vi "TCL Open BaseFile.vi"() -> (0 "error out":errorcluster, 1 "Event File Refnum":refnum<k1>)   [LabVIEW 2009]
uses:
  TCL Global.vi
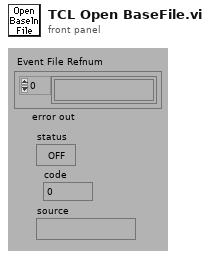
[diagram p1: front panel]
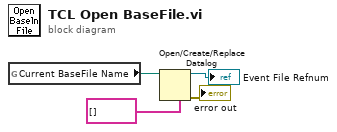
[diagram p0: block diagram]
diagram:
  n1 = global read "TCL Global.vi" "Current BaseFile Name"() -> (w2:path)
  n2 = Open/Create/Replace Datalog(5:string[] [], 11:w2) -> (0:→"error out":errorcluster, 3:→"Event File Refnum":refnum<k1>)  [unwired: 4 in, 1 out]
